vi "File Management.vi"(7 "Operation (1: Export Data Log)":i32(ring)=1 items=["Delete File", "Export Data Log"], 8 "error in (no error)":errorcluster {"code" format="%.0x"}, 9 "File Location (0: Internal)":i32(ring) items=["Internal", "External"], 10 "File Path":string, 11 "VISA resource name":refnum<visa-resource-name>) -> (0 "error out":errorcluster {"code" format="%.0x"}, 3 "VISA resource name out":refnum<visa-resource-name>)   [LabVIEW 2010, in "Agilent N6700 Series.lvlib"]
doc: "This VI exports a data log file to the external memory port and deletes files.\n\n<b>Note:</b>\n\nThis VI only applies to the N6705B DC Power Analyzer."
uses:
  Agilent N6700 Series.lvlib
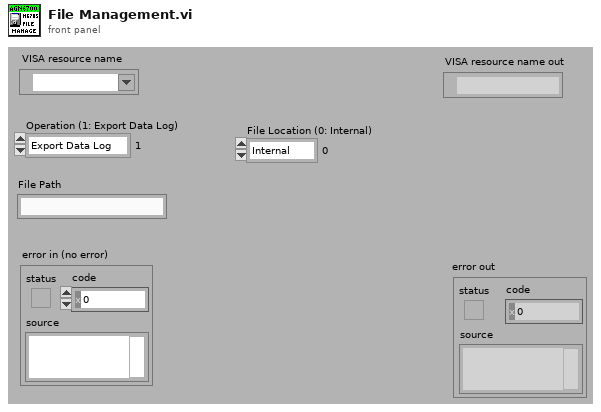
[diagram p1: front panel]
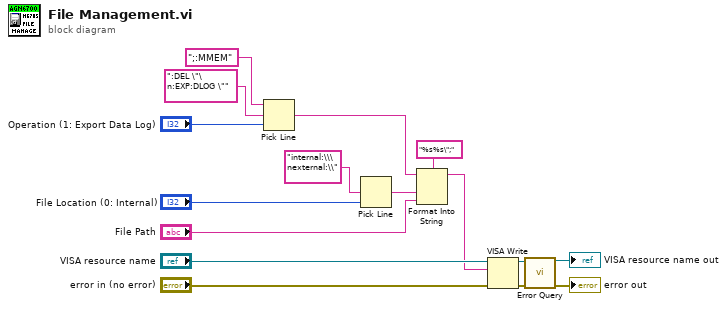
[diagram p0: block diagram]
diagram:
  n1 = Pick Line(string ("")=";:MMEM", multi-line string=":DEL \"\n:EXP:DLOG \"", line index="Operation (1: Export Data Log)") -> (output string=w6:string)
  n2 = Pick Line(multi-line string="internal:\\\nexternal:\\", line index="File Location (0: Internal)") -> (output string=w1:string)  [unwired: 1 in]
  n3 = Format Into String(format string="%s%s\";", initial string=w6, w1, "File Path") -> (resulting string=w5:string)  [unwired: 1 in, 1 out]
  n4 = VISA Write(VISA resource name="VISA resource name", write buffer=w5, error in (no error)="error in (no error)") -> (VISA resource name out=w12:refnum<visa-resource-name>, error out=w11:errorcluster)  [unwired: 1 out]
  n5 = call "Error Query.vi"("VISA resource name"=w12, "error in (no error)"=w11) -> ("VISA resource name out"=→"VISA resource name out":refnum<visa-resource-name>, "error out"=→"error out":errorcluster)  [unwired: 10 in, 2 out]
